vi "Save Batch to DB.vi"(8 "error in":errorcluster, 10 "GTron DB":path=path "D:/SQL Database/Gtron Database.db", 11 "Values":string[][](array[string])) -> (0 "error out":errorcluster)   [LabVIEW 2019, in "DataLogger.lvclass"]
doc: "Save batch Details"
uses:
  DataLogger.lvclass
  <vilib>/drjdpowell/SQLite Library/SQL Connection/Open (path).vi
  <vilib>/drjdpowell/SQLite Library/SQL Connection/Connection.lvclass
  <vilib>/drjdpowell/SQLite Library/SQL Statement/SQL Statement.lvclass
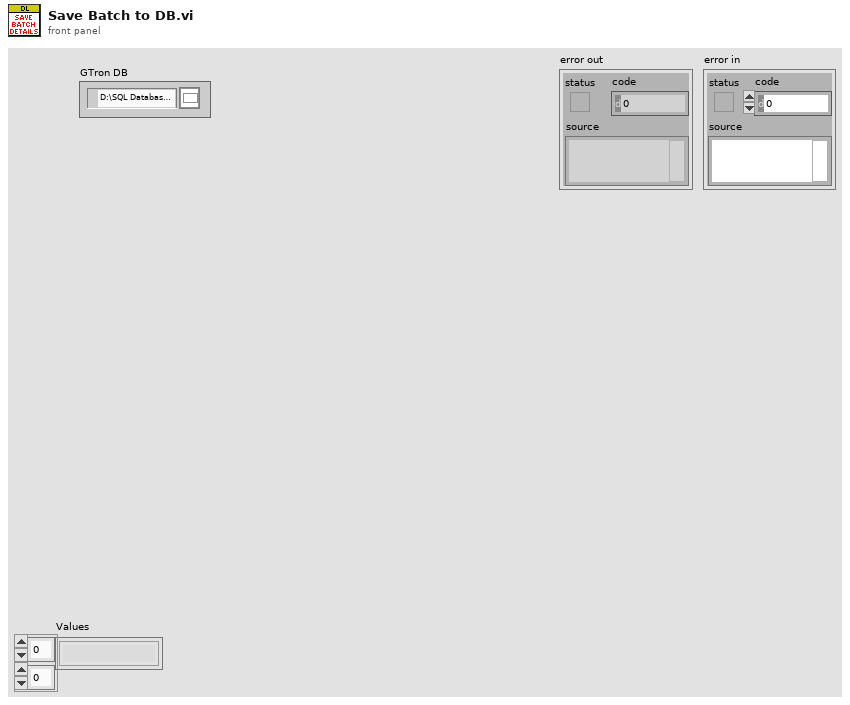
[diagram p1: front panel]
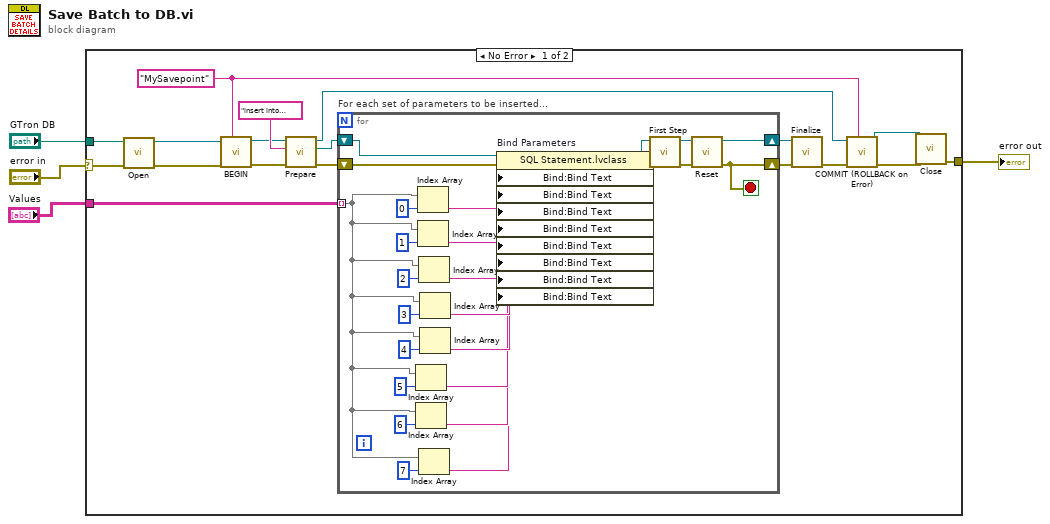
[diagram p0: block diagram]
diagram:
  n1 = case shown="No Error" "error in" {
    selector: "error in" -> [w6 w48]
    tunnel: "GTron DB" -> [w10 _]
    tunnel: [w9 w48] -> w3
    tunnel: "Values" -> [w5 _]
    frame No Error {
      w13 = "MySavepoint" ("Savepoint name")
      n2 = call-poly <vilib>:"Open.vi"("error in (no error)"=w6, "db file"=w10) -> ("error out"=w22:errorcluster, "SQLite Connection"=w21:refnum<class "Connection.lvclass">)  [unwired: 8 in]
      n3 = call <vilib>:"BEGIN.vi"("Savepoint name"=w13, "error in (no error)"=w22, "Connection in"=w21) -> ("error out"=w14:errorcluster, "Connection out"=w15:refnum<class "Connection.lvclass">)  [unwired: 7 in]
      n4 = call <vilib>:"Prepare.vi"("error in (no error)"=w14, "SQL"="insert into BatchDetails  VALUES (?,?,?,?,?,?,?,?)" ("INSERT statement"), "SQLite Connection in"=w15) -> ("error out"=w19:errorcluster, "SQL Statement"=w20:refnum<class "SQL Statement.lvclass">, "SQLite Connection"=w12:refnum<class "Connection.lvclass">)  [unwired: 4 in, 2 out]
      n5 = for "For each set of parameters to be inserted..." {
        shift-right: [w45] -> w17
        shift-left: w20 -> [w47]
        shift-right: [w44] -> w16
        shift-left: w19 -> [w46]
        tunnel: w5 -> [w25] mode=indexing
        stop <- w44 stop-if-true
        n6 = Index Array(array=w25, index=5) -> (element=w27:string)
        n7 = Index Array(array=w25, index=6) -> (element=w26:string)
        n8 = Index Array(array=w25, index=0) -> (element=w32:string)
        n9 = Index Array(array=w25, index=1) -> (element=w31:string)
        n10 = Index Array(array=w25, index=2) -> (element=w30:string)
        n11 = Index Array(array=w25, index=7) -> (element=w23:string)
        n12 = Index Array(array=w25, index=3) -> (element=w29:string)
        n13 = Index Array(array=w25, index=4) -> (element=w28:string)
        n14 = property on="Bind Parameters" class="SQL Statement.lvclass"(reference=w47, error in=w46, "Bind:Bind Text"=w32, "Bind:Bind Text"=w31, "Bind:Bind Text"=w30, "Bind:Bind Text"=w29, "Bind:Bind Text"=w28, "Bind:Bind Text"=w27, "Bind:Bind Text"=w26, "Bind:Bind Text"=w23) -> (reference out=w43:refnum<class "SQL Statement.lvclass">, error out=w42:errorcluster)
        n15 = call <vilib>:"First Step.vi"("error in (no error)"=w42, "SQL Statement in"=w43) -> ("error out"=w41:errorcluster, "SQL Statement"=w40:refnum<class "SQL Statement.lvclass">)  [unwired: 7 in, 1 out]
        n16 = call <vilib>:"Reset.vi"("error in (no error)"=w41, "SQL Statement in"=w40) -> ("error out"=w44:errorcluster, "SQL Statement"=w45:refnum<class "SQL Statement.lvclass">)  [unwired: 8 in]
      }
      n17 = call <vilib>:"Finalize.vi"("error in (no error)"=w16, "SQL Statement in"=w17) -> ("error out"=w11:errorcluster)  [unwired: 9 in]
      n18 = call <vilib>:"COMMIT (ROLLBACK on Error).vi"("Savepoint name"=w13, "error in (no error)"=w11, "Connection in"=w12) -> ("error out"=w7:errorcluster, "Connection out"=w8:refnum<class "Connection.lvclass">)  [unwired: 7 in]
      n19 = call-dynamic "Close.vi"("error in (no error)"=w7, "SQLite Connection in"=w8) -> ("error out"=w9:errorcluster)  [unwired: 9 in]
    }
    frame Error {
    }
  }
  "error out" <- w3
